vi "DB Tools Fetch Next Recordset.vi"   [LabVIEW 2017, in "NI_Database_API.lvlib"]
doc: "Retrieves the next recordset in a multi-recordset query identified by <B>recordset reference</B>. When the current recordset is no longer available, the <B>recordset reference</B> is redirected to the new recordset. Wire data to the reference input to determine the polymorphic instance to use or manually select the instance."
uses:
  <vilib>/addons/database/NI_Database_API.lvlib
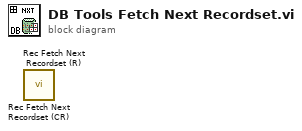
[diagram p0: block diagram]
diagram:
  n1 = call <vilib>:"Rec Fetch Next Recordset (CR).vi"() -> ()  [unwired: 6 in, 2 out]
  n2 = call <vilib>:"Rec Fetch Next Recordset (R).vi"() -> ()  [unwired: 6 in, 2 out]
